vi "Find Timing Section.vi"(8 "error in":errorcluster, 11 "custom device ref":T1 format="%.0x") -> (0 "error out":errorcluster, 2 "timing":T1 format="%.0x", 3 "custom device ref out":T1 format="%.0x")   [LabVIEW 2020, in "AIM ARINC 429 Scripting.lvlib"]
doc: "Returns the <b>logging</b> section of the AIM ARINC 429 custom device."
uses:
  AIM ARINC 429 Scripting.lvlib
  <vilib>/NI VeriStand/Custom Device API/Custom Device Item Ref.ctl
  Constants.vi
  <vilib>/NI VeriStand/Custom Device Tools/Custom Device Utility Library/NI VeriStand - Search for Item by GUID.vi
  <vilib>/NI VeriStand/Custom Device Tools/Custom Device Utility Library/Custom Device Utility Library.lvlib
  <vilib>/NI VeriStand/Custom Device API/Custom Device API.lvlib
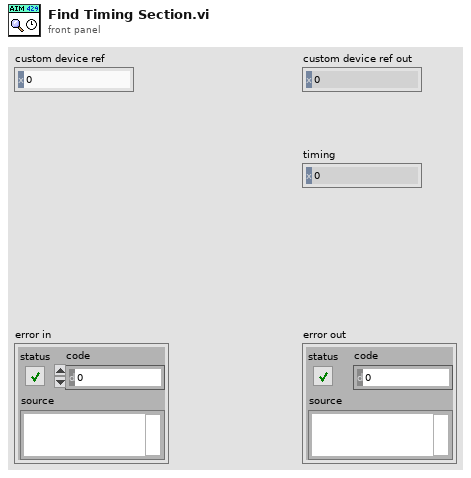
[diagram p1: front panel]
types:
  T1 = typedef "Custom Device API.lvlib/Custom Device Item Ref.ctl" = u64
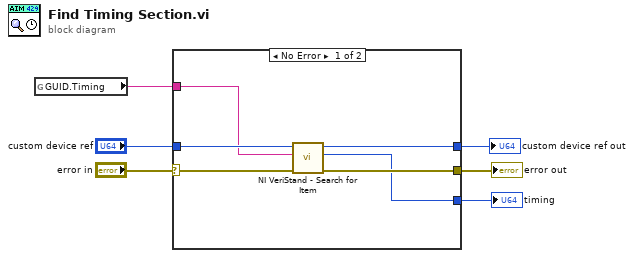
[diagram p0: block diagram]
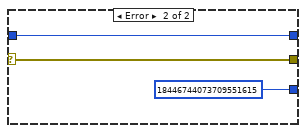
[diagram p2: hidden frame]
diagram:
  n1 = global read "Constants.vi" "GUID.Timing"() -> (w5:string)
  n2 = case shown="No Error" "error in" {
    selector: "error in" -> [w7 w14]
    tunnel: "custom device ref" -> [w12 w15]
    tunnel: w5 -> [w11 _]
    tunnel: [w10 w14] -> w4
    tunnel: [w9 w15] -> w3
    tunnel: [w8 T1 18446744073709551615 ("Item Ref")] -> w2
    frame No Error {
      n3 = call-poly <vilib>:"NI VeriStand - Search for Item.vi"("error in"=w7, "Item GUID"=w11, "Section Ref in"=w12) -> ("error out"=w10:errorcluster, "Item Ref"=w8:T1, "Section Ref out"=w9:T1)  [unwired: 5 in, 1 out]
    }
    frame Error {
    }
  }
  "timing" <- w2
  "error out" <- w4
  "custom device ref out" <- w3
